vi "FlatToRichcif_plugincore_GetOverridesResponse.vi"(5 "OutputClusterType":T1, 11 "InputCluster":T4) -> (3 "OutputCluster":T1)   [LabVIEW 2021, in "CIFCorePlugin_client.lvlib"]
uses:
  CIFCorePlugin_client.lvlib
  cif_plugincore_GetOverridesResponse_Flat.ctl
  cif_plugincore_PluginOverrides_Flat.ctl
  cif_plugincore_TimingOverrides_Flat.ctl
  cif_plugincore_GetOverridesResponse.ctl
  cif_plugincore_PluginOverrides.ctl
  cif_plugincore_TimingOverrides.ctl
  FlatToRichcif_plugincore_TimingOverrides.vi
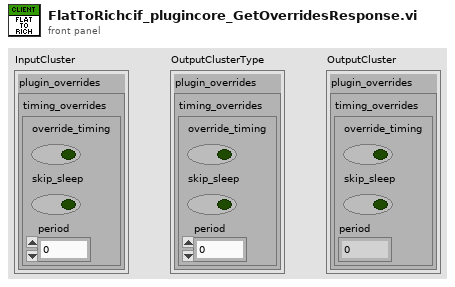
[diagram p1: front panel]
types:
  T1 = typedef "CIFCorePlugin_client.lvlib/cif_plugincore_GetOverridesResponse.ctl" = cluster{"plugin_overrides":T2}
  T2 = typedef "CIFCorePlugin_client.lvlib/cif_plugincore_PluginOverrides.ctl" = cluster{"timing_overrides":T3}
  T3 = typedef "CIFCorePlugin_client.lvlib/cif_plugincore_TimingOverrides.ctl" = cluster{"override_timing":bool, "skip_sleep":bool, "period":dbl}
  T4 = typedef "CIFCorePlugin_client.lvlib/cif_plugincore_GetOverridesResponse_Flat.ctl" = cluster{"plugin_overrides":T5}
  T5 = typedef "CIFCorePlugin_client.lvlib/cif_plugincore_PluginOverrides_Flat.ctl" = cluster{"timing_overrides":T6}
  T6 = typedef "CIFCorePlugin_client.lvlib/cif_plugincore_TimingOverrides_Flat.ctl" = cluster{"override_timing":bool, "skip_sleep":bool, "period":dbl}
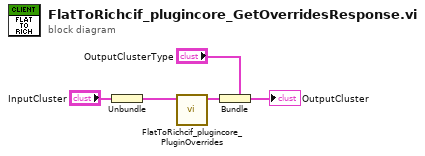
[diagram p0: block diagram]
diagram:
  n1 = Unbundle "Unbundle"("InputCluster") -> ("plugin_overrides"=w2:T5)
  n2 = call "FlatToRichcif_plugincore_PluginOverrides.vi"("InputCluster"=w2) -> ("OutputCluster"=w1:T2)  [unwired: 10 in]
  n3 = Bundle "Bundle"(cluster="OutputClusterType", "plugin_overrides"=w1) -> (→"OutputCluster":T1)
